vi "print_document.vi"(8 "error in (no error)":errorcluster, 10 "IReport in":refnum<class "IReport.lvclass">, 11 "Printer in":refnum<class "Printer.lvclass">) -> (0 "error out":errorcluster, 3 "Printer out":refnum<class "Printer.lvclass">)   [LabVIEW 2024, in "Printer.lvclass"]
uses:
  Printer.lvclass
  Printer.lvclass/Printer.ctl
  IReport/IReport.lvclass
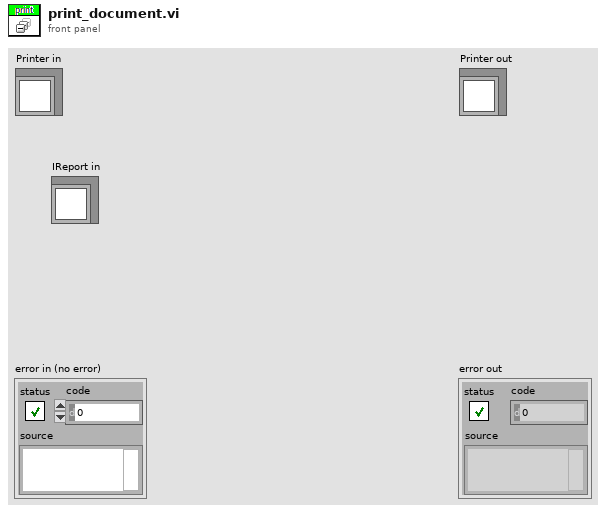
[diagram p1: front panel]
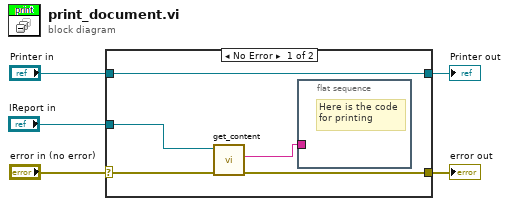
[diagram p0: block diagram]
diagram:
  n1 = case shown="No Error" "error in (no error)" {
    selector: "error in (no error)" -> [w9 w12]
    tunnel: [w8 w12] -> w4
    tunnel: [w10 w11] -> w2
    tunnel: "Printer in" -> [w10 w11]
    tunnel: "IReport in" -> [w6 _]
    frame No Error {
      n2 = call-dynamic "get_content.vi"("error in (no error)"=w9, "IDocument in"=w6) -> ("error out"=w8:errorcluster, "String"=w7:string)  [unwired: 7 in, 1 out]
      n3 = flat-sequence {
        tunnel: w7 -> [_]
        frame #0 {
          # "Here is the code\nfor printing"
        }
      }
    }
    frame Error {
    }
  }
  "error out" <- w4
  "Printer out" <- w2
